vi "generador_4channel_sub.vi"(4 "A":dbl, 5 "Ring":T1, 6 "t1":dbl, 7 "N":dbl, 8 "t0":dbl, 9 "T":dbl, 10 "i":dbl) -> (3 "Waveform Chart":dbl(graph)=1.0)   [LabVIEW 2011]
uses:
  Control 1.ctl
  <vilib>/gmath/NI_Gmath.lvlib
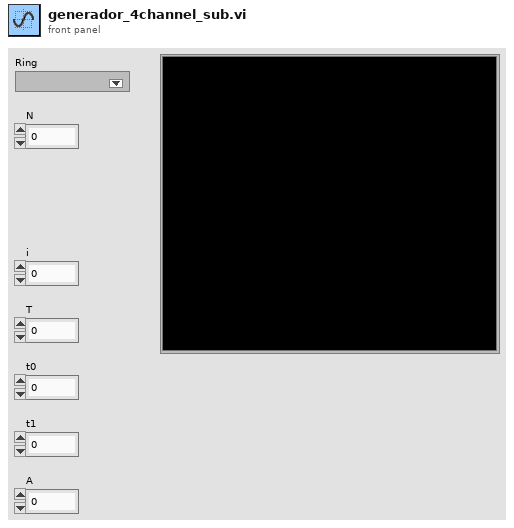
[diagram p1: front panel]
types:
  T1 = typedef "Control 1.ctl" = u16
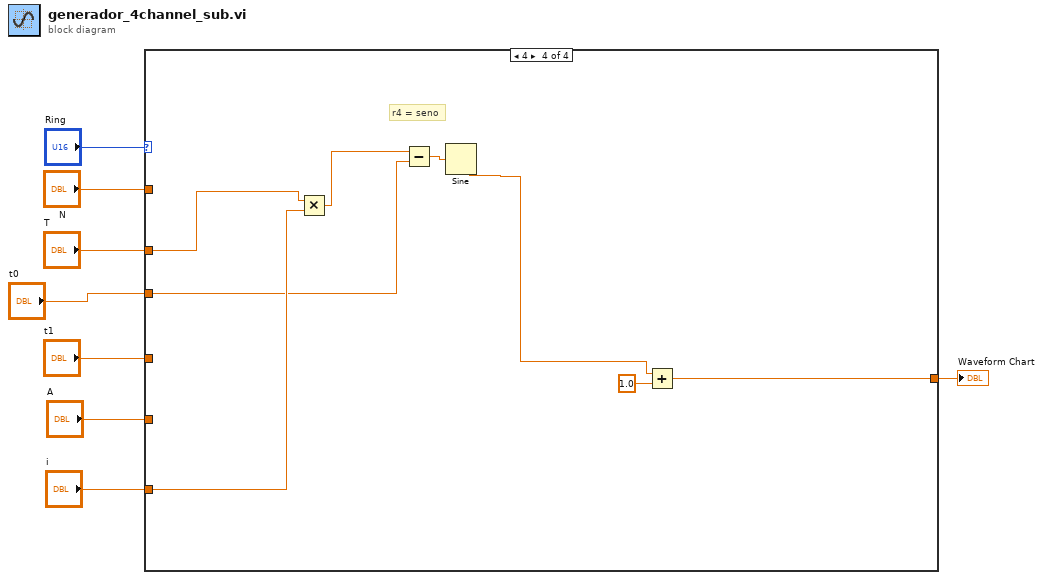
[diagram p0: block diagram]
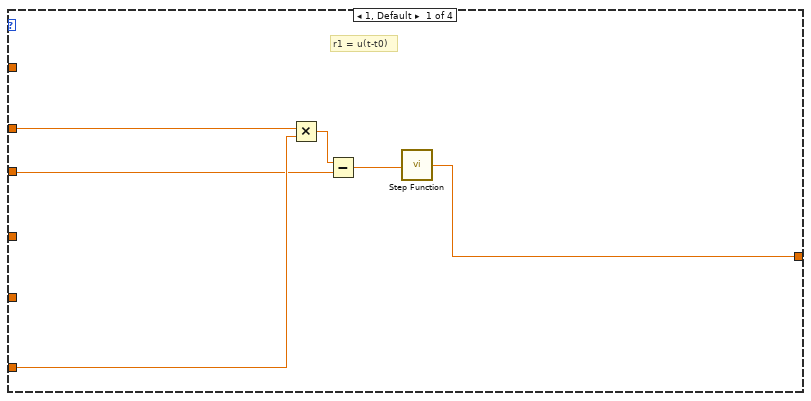
[diagram p2: hidden frame]
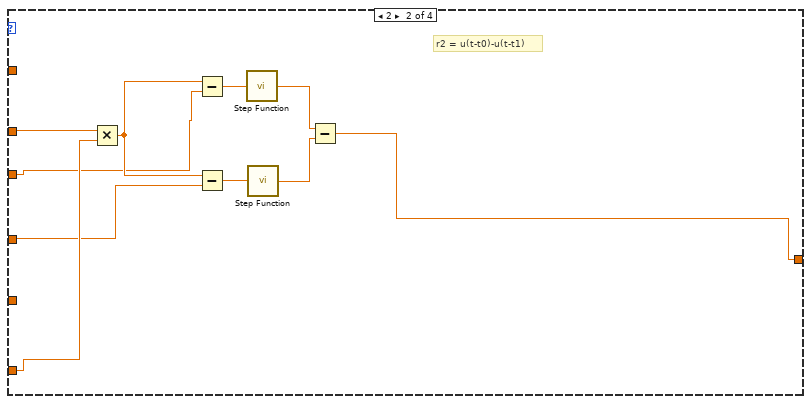
[diagram p3: hidden frame]
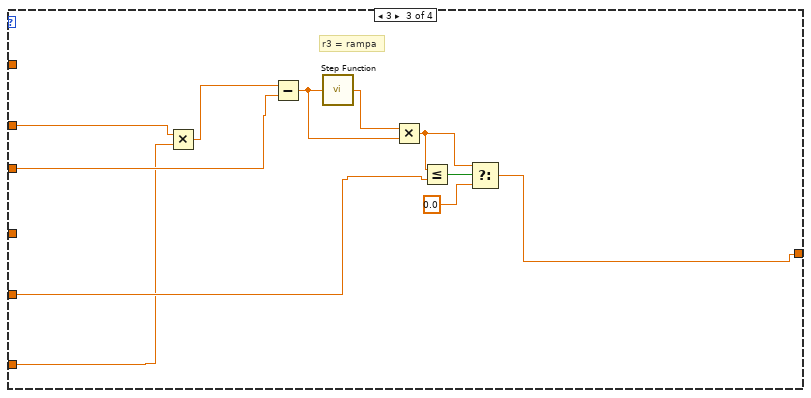
[diagram p4: hidden frame]
diagram:
  n1 = case shown="4" "Ring" {
    tunnel: "N" -> [_ _ _ _]
    tunnel: "T" -> [w10 w19 w29 w39]
    tunnel: "t0" -> [w11 w17 w28 w40]
    tunnel: "t1" -> [_ w16 _ _]
    tunnel: "A" -> [_ _ w27 _]
    tunnel: "i" -> [w12 w18 w26 w41]
    tunnel: [w9 w15 w25 w36] -> w1
    frame 1, Default {
      # "r1 = u(t-t0)"
      n2 = Multiply(x=w10, y=w12) -> (x*y=w14:dbl)
      n3 = Subtract(x=w14, y=w11) -> (x-y=w13:dbl)
      n4 = call <vilib>:"Step Function.vi"("x"=w13) -> ("step(x)"=w9:dbl)
    }
    frame 2 {
      # "r2 = u(t-t0)-u(t-t1)"
      n5 = Multiply(x=w19, y=w18) -> (x*y=w20:dbl)
      n6 = Subtract(x=w20, y=w17) -> (x-y=w21:dbl)
      n7 = Subtract(x=w20, y=w16) -> (x-y=w22:dbl)
      n8 = call <vilib>:"Step Function.vi"("x"=w21) -> ("step(x)"=w23:dbl)
      n9 = call <vilib>:"Step Function.vi"("x"=w22) -> ("step(x)"=w24:dbl)
      n10 = Subtract(x=w23, y=w24) -> (x-y=w15:dbl)
    }
    frame 3 {
      # "r3 = rampa"
      n11 = Multiply(x=w29, y=w26) -> (x*y=w33:dbl)
      n12 = Subtract(x=w33, y=w28) -> (x-y=w34:dbl)
      n13 = call <vilib>:"Step Function.vi"("x"=w34) -> ("step(x)"=w30:dbl)
      n14 = Multiply(x=w30, y=w34) -> (x*y=w32:dbl)
      n15 = Less Or Equal?(x=w32, y=w27) -> (x <= y?=w31:bool)
      n16 = Select(t=w32, s=w31, f=0.0) -> (s? t:f=w25:dbl)
    }
    frame 4 {
      # "r4 = seno"
      n17 = Multiply(x=w39, y=w41) -> (x*y=w42:dbl)
      n18 = Subtract(x=w42, y=w40) -> (x-y=w43:dbl)
      n19 = Sine(x=w43) -> (sin(x)=w37:dbl)
      n20 = Add(x=w37, y=1.0) -> (x+y=w36:dbl)
    }
  }
  "Waveform Chart" <- w1
